vi "Cycle.vi"(8 "error in (no error)":errorcluster, 11 "PassiveExperiment In":refnum<class "PassiveExperiment.lvclass">) -> (0 "error out":errorcluster, 3 "PassiveExperiment Out":refnum<class "PassiveExperiment.lvclass">)   [LabVIEW 2014, in "AcquisitionCoreObjects.lvlib" / "PassiveExperiment.lvclass"]
uses:
  PassiveExperiment.lvclass
  MatlabExperiment/MatlabExperiment.lvclass
panel:
  out "XY Graph":cluster{"horizontal":dbl[], "vertical":dbl[]}[](graph)
  out "ExperimentStats":T1
  in  "FixationRadius":dbl=34.0
  in  "RewardAmount":dbl=50.0
  out "Timeouts":T2={"Intertrial"=1500.0, "AcquireFixation"=4000.0, "HoldFixation"=300.0, "DelayPeriod"=2000.0, "ResponsePeriod"=0.0}
  in  "Eye Params":dbl[](array[numeric])
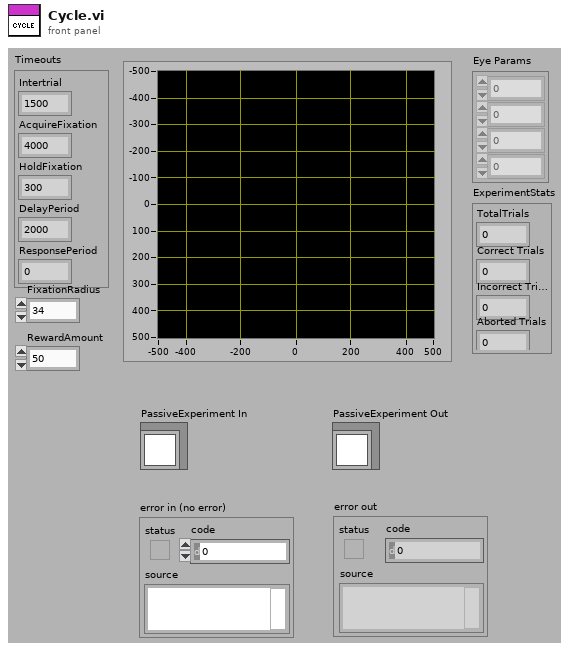
[diagram p1: front panel]
types:
  T1 = cluster{"TotalTrials":dbl, "Correct Trials":dbl, "Incorrect Trials":dbl, "Aborted Trials":dbl}
  T2 = cluster{"Intertrial":dbl, "AcquireFixation":dbl, "HoldFixation":dbl, "DelayPeriod":dbl, "ResponsePeriod":dbl}
  T3 = cluster{"TotalTrials":u32, "Correct Trials":u32, "Incorrect Trials":u32, "Aborted Trials":u32}
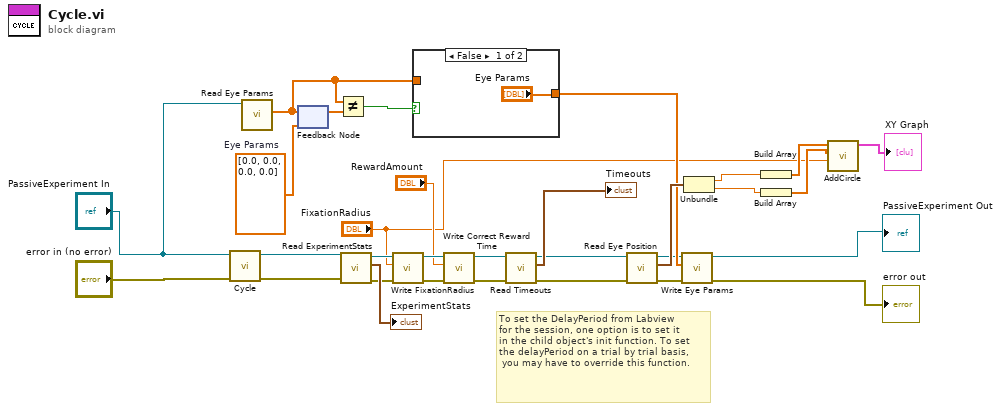
[diagram p0: block diagram]
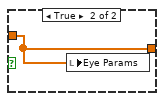
[diagram p2: hidden frame]
diagram:
  w25 = dbl[] [0.0, 0.0, 0.0, 0.0]  # Eye Params
  # "To set the DelayPeriod from Labview\nfor the session, one option is to set it \nin the child object's init function. To set\nthe delayPeriod on a trial by trial basis,\n you may have to override this function."
  n1 = call-parent "Cycle.vi"("error in (no error)"="error in (no error)", "MatlabExperiment In"="PassiveExperiment In") -> ("error out"=w5:errorcluster, "MatlabExperiment Out"=w6:refnum<class "PassiveExperiment.lvclass">)  [unwired: 8 in]
  n2 = call-dynamic "Read Eye Params.vi"("TrialBasedExperiment in"="PassiveExperiment In") -> ("Eye Params"=w26:dbl[])  [unwired: 8 in, 2 out]
  n3 = feedback #1(w25) -> (w23:dbl[])
  n4 = feedback-in #1(w26) -> ()
  n5 = Not Equal?(x=w26, y=w23) -> (x != y?=w24:bool)
  n6 = call-dynamic "Read ExperimentStats.vi"("error in (no error)"=w5, "TrialBasedExperiment in"=w6) -> ("error out"=w15:errorcluster, "ExperimentStats"=→"ExperimentStats":T3, "TrialBasedExperiment out"=w14:refnum<class "PassiveExperiment.lvclass">)  [unwired: 7 in]
  n7 = call-dynamic "Write FixationRadius.vi"("error in (no error)"=w15, "FixationRadius"="FixationRadius", "MatlabExperiment in"=w14) -> ("error out"=w18:errorcluster, "MatlabExperiment out"=w17:refnum<class "PassiveExperiment.lvclass">)  [unwired: 7 in]
  n8 = case shown="False" w24 {
    tunnel: ["Eye Params" w33] -> w29
    tunnel: w26 -> [_ w33]
    frame False {
    }
    frame True {
      n9 = local write "Eye Params"(w33) -> ()
    }
  }
  n10 = call-dynamic "Write Correct Reward Time.vi"("error in (no error)"=w18, "Correct Reward Time"="RewardAmount", "MatlabExperiment in"=w17) -> ("error out"=w20:errorcluster, "MatlabExperiment out"=w19:refnum<class "PassiveExperiment.lvclass">)  [unwired: 7 in]
  n11 = call-dynamic "Read Timeouts.vi"("error in (no error)"=w20, "TrialBasedExperiment in"=w19) -> ("error out"=w21:errorcluster, "Timeouts"=→"Timeouts":T2, "TrialBasedExperiment out"=w1:refnum<class "PassiveExperiment.lvclass">)  [unwired: 7 in]
  n12 = call-dynamic "Read Eye Position.vi"("error in (no error)"=w21, "TrialBasedExperiment in"=w1) -> ("error out"=w28:errorcluster, "Eye Position"=w30:cluster{"Horizontal":dbl, "Vertical":dbl}, "TrialBasedExperiment out"=w27:refnum<class "PassiveExperiment.lvclass">)  [unwired: 7 in]
  n13 = call-dynamic "Write Eye Params.vi"("error in (no error)"=w28, "Eye Params"=w29, "TrialBasedExperiment in"=w27) -> ("error out"=→"error out":errorcluster, "TrialBasedExperiment out"=→"PassiveExperiment Out":refnum<class "PassiveExperiment.lvclass">)  [unwired: 7 in]
  n14 = Unbundle(w30) -> ("Horizontal"=w13:dbl, "Vertical"=w12:dbl)
  n15 = Build Array(w13) -> (w11:dbl[])
  n16 = Build Array(w12) -> (w10:dbl[])
  n17 = call "AddCircle.vi"("radius"="FixationRadius", "vertical"=w10, "horizontal"=w11) -> ("output"=→"XY Graph":cluster{"horizontal":dbl[], "vertical":dbl[]}[])  [unwired: 8 in]
